vi "Percent-IPS.vi"(2 "Numeric":dbl) -> ()   [LabVIEW 2011]
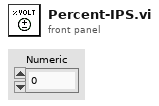
[diagram p1: front panel]
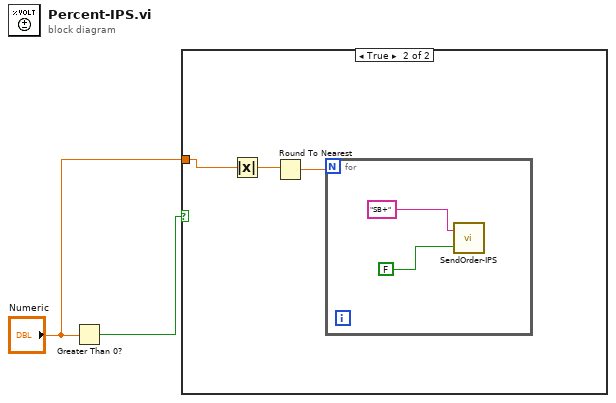
[diagram p0: block diagram]
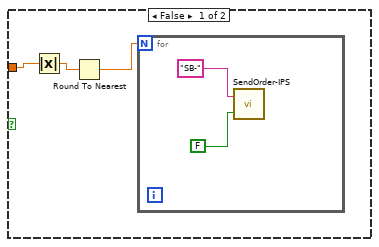
[diagram p2: hidden frame]
diagram:
  n1 = Greater Than 0?(x="Numeric") -> (x > 0?=w2:bool)
  n2 = case shown="True" w2 {
    tunnel: "Numeric" -> [w5 w10]
    frame False {
      n3 = Absolute Value(x=w5) -> (abs(x)=w4:dbl)
      n4 = Round To Nearest(number=w4) -> (nearest integer value=w3:dbl)
      n5 = for {
        N: w3 -> [_]
        n6 = call "SendOrder-IPS.vi"("read"=FALSE, "string to write"="SB-") -> ()  [unwired: 1 out]
      }
    }
    frame True {
      n7 = Absolute Value(x=w10) -> (abs(x)=w9:dbl)
      n8 = Round To Nearest(number=w9) -> (nearest integer value=w8:dbl)
      n9 = for {
        N: w8 -> [_]
        n10 = call "SendOrder-IPS.vi"("read"=FALSE, "string to write"="SB+") -> ()  [unwired: 1 out]
      }
    }
  }
